vi "constructor.vi"(10 "Beverage.lvclass":refnum<class "Beverage.lvclass">, 11 "Whip in":refnum<class "Whip.lvclass">) -> (3 "Whip out":refnum<class "Whip.lvclass">)   [LabVIEW 2020, in "Whip.lvclass"]
uses:
  Whip.lvclass
  Beverage.lvclass
  Whip.lvclass/Whip.ctl
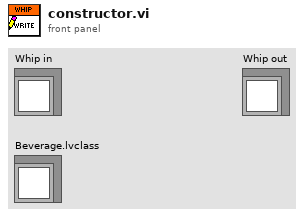
[diagram p1: front panel]
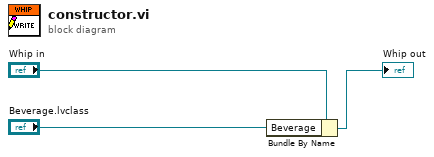
[diagram p0: block diagram]
diagram:
  n1 = Bundle By Name(cluster="Whip in", "Beverage"="Beverage.lvclass") -> (→"Whip out":refnum<class "Whip.lvclass">)
